vi "Init DaqEngine local AI SM.vi"(7 "AI TaskName":string, 8 "error in (no error)":errorcluster, 11 "DAQ Process AppData":T1) -> (0 "error out":errorcluster, 1 "local LoopCmdQ":refnum<queue>, 3 "DaqProces AI AppData+":T12)   [LabVIEW 2017, in "DAQ.lvclass"]
doc: "Developed by Kevin Thompson\nkevin@thompsonengineering.net\n\nCopyright 2018-2020\nThompson Engineering, LLC"
uses:
  DAQ.lvclass
  Process_DAQ SM AppData--cluster.ctl
  DataTypes/TD DAQ Settings--cluster.ctl
  DataTypes/TD DI Instrument Settings--cluster.ctl
  DataTypes/TD AI Instrument Settings--cluster.ctl
  DataTypes/TD AI InstSettings--cluster.ctl
  TD SimAI Ranges--cluster.ctl
  <vilib>/TELLC/Dynamic CVT API/TD Dynamic CVT DVR--ref.ctl
  DataTypes/TD AI local thread params--clustser.ctl
  Support/DataQueues/DataTypes/Analog DataSet MultiRow--QRef.ctl
  Support/DataQueues/DataTypes/Analog DataSet MultiRow--cluster.ctl
  Support/DataQueues/DataTypes/Analog DataSet MultiRow & ChanNames--QRef.ctl
  Support/DataQueues/DataTypes/Analog DataSet MultiRow & ChanNames--cluster.ctl
  DataTypes/TD AI TaskIO.ctl
  Support/DataQueues/DataTypes/DataQ SelectType--enum.ctl
  DAQ.lvclass/DAQ.ctl
  Accessors/Get DAQNodes Dict.vi
  Accessors/Get DAQ Settings.vi
  Accessors/Get Dependency.vi
  Get AI DAQ SMQ - single.vi
  Config/Config.lvclass
  Support/DataQueues/DataQueues.lvclass
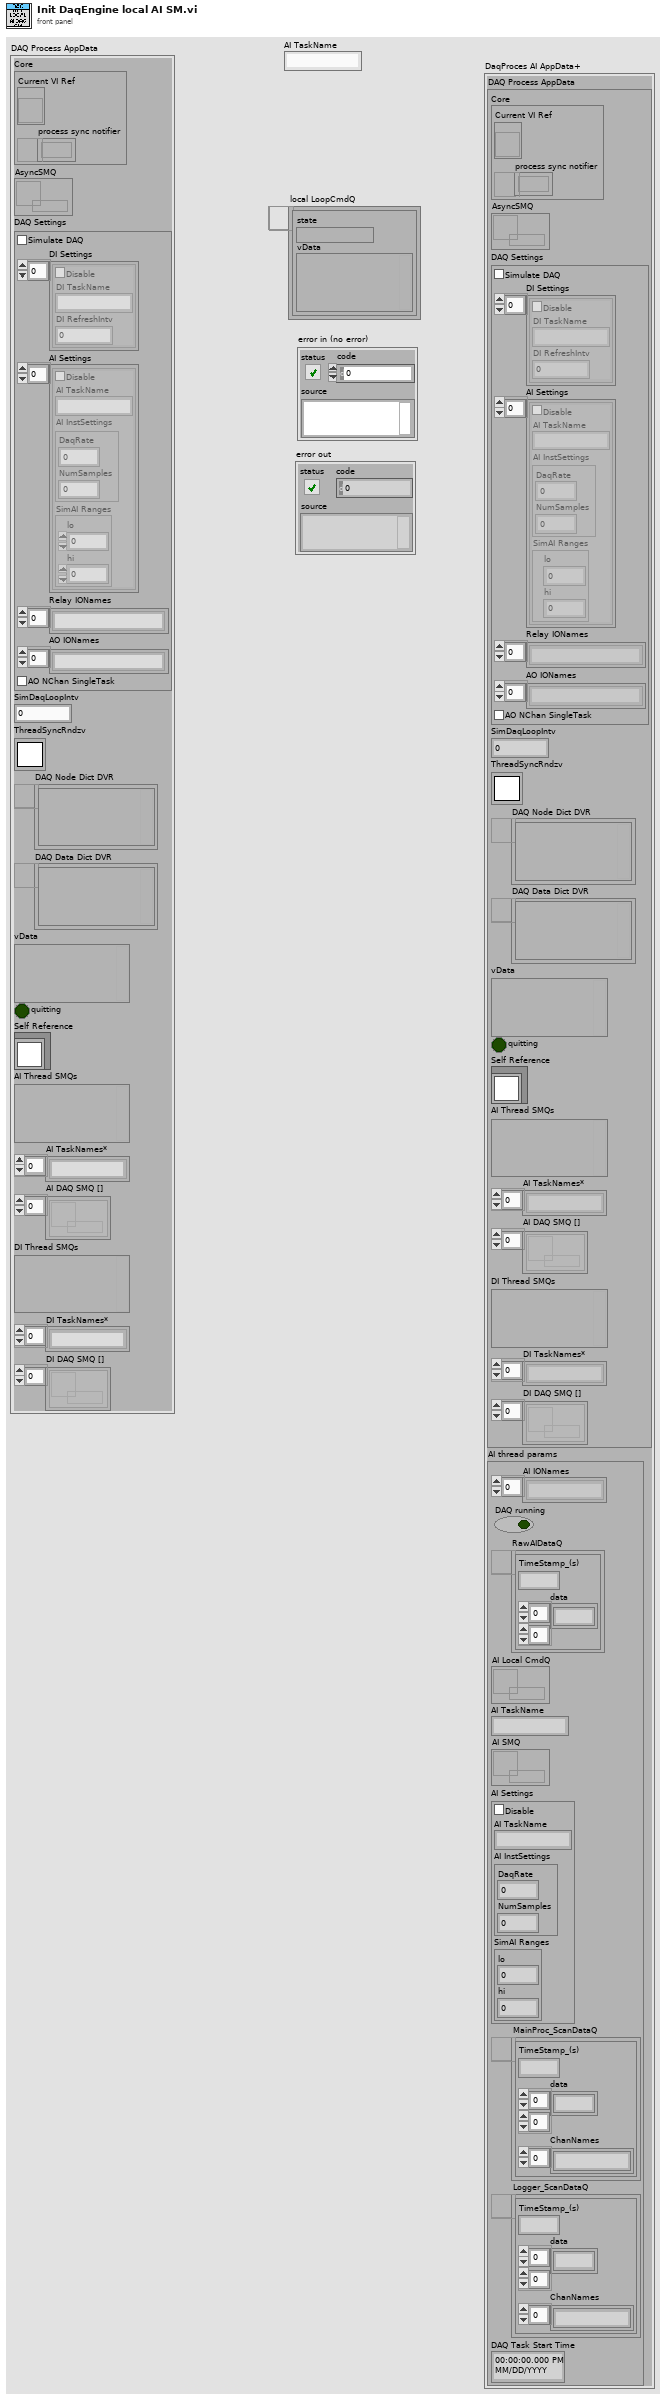
[diagram p1: front panel]
types:
  T1 = typedef "DAQ.lvclass/Process_DAQ SM AppData--cluster.ctl" = cluster{"Core":cluster{"Current VI Ref":refnum<vi>, "process sync notifier":refnum<notifier>}, "AsyncSMQ":refnum<queue>, "DAQ Settings":T2, "SimDaqLoopIntv":i32, "ThreadSyncRndzv":T7, "DAQ Node Dict DVR":T8, "DAQ Data Dict DVR":T8, "vData":variant, "quitting":bool, "Self Reference":refnum<class "DAQ.lvclass">, "AI Thread SMQs":variant, "AI TaskNames*":string[], "AI DAQ SMQ []":refnum<queue>[], "DI Thread SMQs":variant, "DI TaskNames*":string[], "DI DAQ SMQ []":refnum<queue>[]}
  T2 = typedef "DAQ.lvclass/TD DAQ Settings--cluster.ctl" = cluster{"Simulate DAQ":bool, "DI Settings":T3[], "AI Settings":T4[], "Relay IONames":string[], "AO IONames":string[], "AO NChan SingleTask":bool}
  T3 = typedef "DAQ.lvclass/TD DI Instrument Settings--cluster.ctl" = cluster{"Disable":bool, "DI TaskName":string, "DI RefreshIntv":i32}
  T4 = typedef "DAQ.lvclass/TD AI Instrument Settings--cluster.ctl" = cluster{"Disable":bool, "AI TaskName":string, "AI InstSettings":T5, "SimAI Ranges":T6}
  T5 = typedef "DAQ.lvclass/TD AI InstSettings--cluster.ctl" = cluster{"DaqRate":dbl, "NumSamples":i32}
  T6 = typedef "DAQ.lvclass/TD SimAI Ranges--cluster.ctl" = cluster{"lo":dbl, "hi":dbl}
  T7 = typedef "Rendezvous RefNum" = refnum<k1>
  T8 = typedef "TD Dynamic CVT DVR--ref.ctl" = refnum<data-value>
  T9 = typedef "DAQ.lvclass/TD AI local thread params--clustser.ctl" = cluster{"AI IONames":string[], "DAQ running":bool, "RawAIDataQ":T10, "AI Local CmdQ":refnum<queue>, "AI TaskName":string, "AI SMQ":refnum<queue>, "AI Settings":T4, "MainProc_ScanDataQ":T11, "Logger_ScanDataQ":T11, "DAQ Task Start Time":timestamp}
  T10 = typedef "DataQueues.lvclass/Analog DataSet MultiRow--QRef.ctl" = refnum<queue>
  T11 = typedef "DataQueues.lvclass/Analog DataSet MultiRow & ChanNames--QRef.ctl" = refnum<queue>
  T12 = cluster{"DAQ Process AppData":T1, "AI thread params":T9}
  T13 = typedef "DataQueues.lvclass/DataQ SelectType--enum.ctl" = enum16{"MainProcess", "LogEngine", "LocalDAQThread"}
  T14 = typedef "DAQ.lvclass/TD AI TaskIO.ctl" = cluster{"AI TaskName":string, "IONames":string[], "DAQmx AI TaskRef":refnum<k21>}
  T15 = typedef "DAQ.lvclass/Dependency--cluster.ctl" = cluster{"Config":refnum<class "Config.lvclass">, "DataQueues":refnum<class "DataQueues.lvclass">}
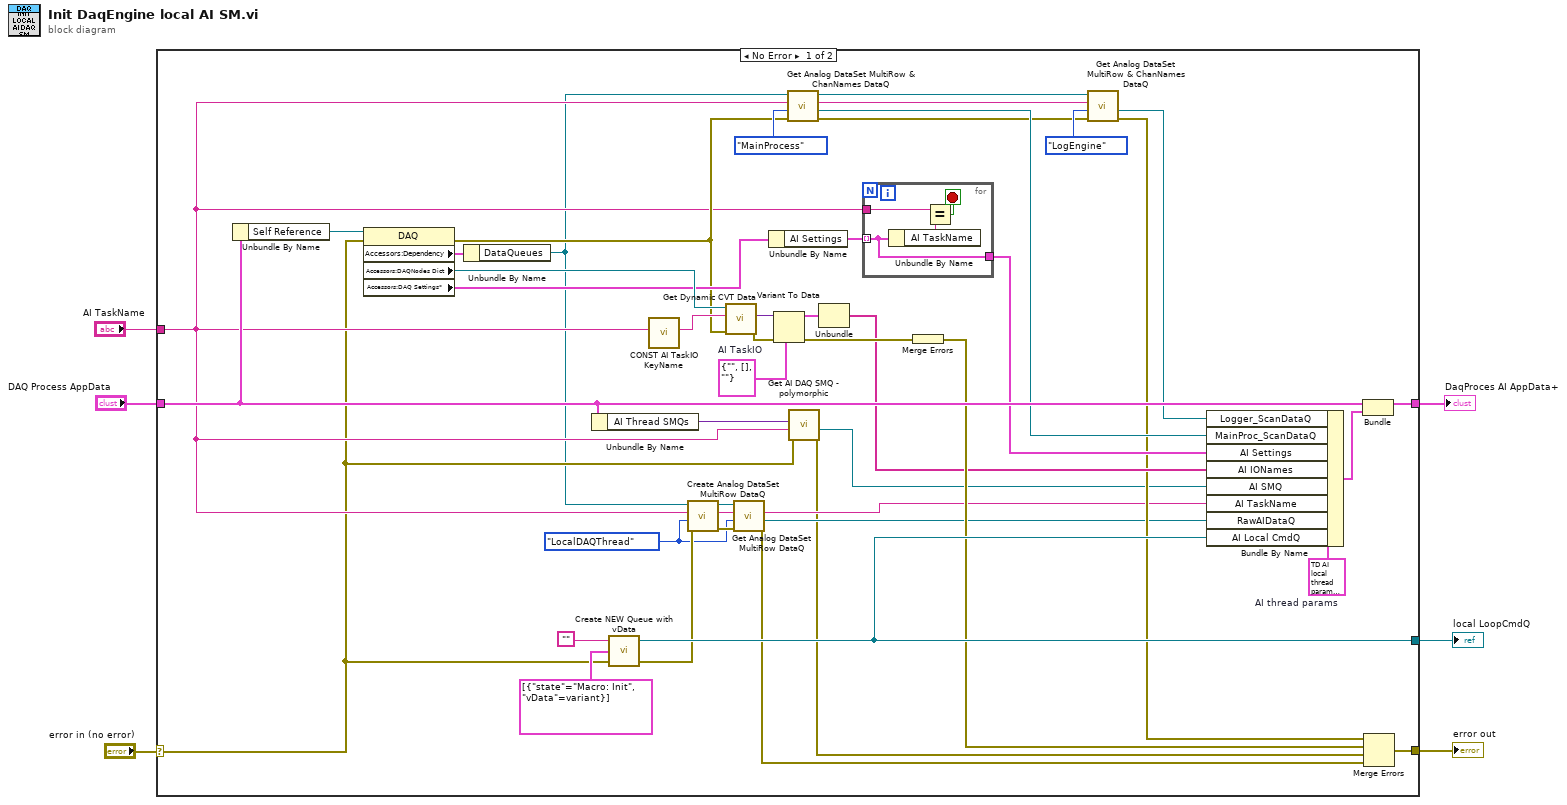
[diagram p0: block diagram]
diagram:
  n1 = case shown="No Error" "error in (no error)" {
    selector: "error in (no error)" -> [w11 w56]
    tunnel: "DAQ Process AppData" -> [w40 _]
    tunnel: [w47 _] -> w6
    tunnel: [w49 _] -> w3
    tunnel: [w50 w56] -> w5
    tunnel: "AI TaskName" -> [w13 _]
    frame No Error {
      w9 = DataQ_SelectType--enum."LocalDAQThread" ("Select")
      w32 = T14 {"AI TaskName"="", "IONames"=[], "DAQmx AI TaskRef"=""}  # AI TaskIO
      w48 = T9 {"AI IONames"=[], "DAQ running"=FALSE, "RawAIDataQ"=refnum, "AI Local CmdQ"=refnum, "AI TaskName"="", "AI SMQ"=refnum, "AI Settings"={"Disable"=FALSE, "AI TaskName"="", "AI InstSettings"={"DaqRate"=0.0, "NumSamples"=0}, "SimAI Ranges"={"lo"=0.0, "hi"=0.0}}, "MainProc_ScanDataQ"=refnum, "Logger_ScanDataQ"=refnum, "DAQ Task Start Time"=timestamp(0 s since 1904-01-01)}  # AI thread params
      n2 = Unbundle By Name(w40) -> ("Self Reference"=w46:refnum<class "DAQ.lvclass">)
      n3 = property class="DAQ"(reference=w46, error in=w11) -> (error out=w30:errorcluster, "Accessors:Dependency"=w8:T15, "Accessors:DAQNodes Dict"=w36:T8, "Accessors:DAQ Settings*"=w33:T2)  [unwired: 1 out]
      n4 = Unbundle By Name(w8) -> ("DataQueues"=w7:refnum<class "DataQueues.lvclass">)
      n5 = Unbundle By Name(w40) -> ("AI Thread SMQs"=w14:variant)
      n6 = call <vilib>:"Create NEW Queue with vData.vi"("error in (no error)"=w11, "Initial States"=cluster{"state":string, "vData":variant}[] [{"state"="Macro: Init", "vData"=variant}], "Name (SMQ)"="") -> ("error out"=w15:errorcluster, "queue out"=w47:refnum<queue>)  [unwired: 1 in]
      n7 = call "CONST AI TaskIO KeyName.vi"("AI TaskName"=w13) -> ("AI TaskIO (KeyName)"=w45:string)  [unwired: 10 in]
      n8 = call "Create Analog DataSet MultiRow DataQ.vi"("error in (no error)"=w15, "Select"=w9, "TaskName"=w13, "DataQueues in"=w7) -> ("error out"=w17:errorcluster, "TaskName out"=w18:string, "DataQueues out"=w16:refnum<class "DataQueues.lvclass">)  [unwired: 5 in]
      n9 = call <vilib>:"Get Dynamic CVT Data.vi"("error in (no error)"=w30, "DataName"=w45, "dCVT DVR"=w36) -> ("error out"=w43:errorcluster, "value"=w44:variant)  [unwired: 5 in, 2 out]
      n10 = call "Get Analog DataSet MultiRow DataQ.vi"("error in (no error)"=w17, "Select"=w9, "TaskName"=w18, "DataQueues in"=w16) -> ("error out"=w20:errorcluster, "Analog DataSet MultiRow QRef"=w21:T10, "TaskName out"=w19:string)  [unwired: 3 in, 2 out]
      n11 = Unbundle By Name(w33) -> ("AI Settings"=w39:T4[])
      n12 = Variant To Data(error in=w43, type=w32, Variant=w44) -> (data=w35:T14, error out=w42:errorcluster)
      n13 = call "Get Analog DataSet MultiRow & ChanNames DataQ.vi"("error in (no error)"=w30, "Select"=DataQ_SelectType--enum."MainProcess", "TaskName"=w13, "DataQueues in"=w7) -> ("error out"=w23:errorcluster, "Analog DataSet MultiRow & ChanNames QRef"=w29:T11, "TaskName out"=w26:string, "DataQueues out"=w27:refnum<class "DataQueues.lvclass">)  [unwired: 3 in, 1 out]
      n14 = call-poly "Get AI DAQ SMQ - polymorphic.vi"("error in (no error)"=w11, "AI TaskName"=w13, "AI Thread SMQs"=w14) -> ("error out"=w10:errorcluster, "AI DAQ SMQ"=w12:refnum<queue>)  [unwired: 6 in, 1 out]
      n15 = Unbundle(w35) -> ("IONames"=w34:string[])  [unwired: 2 out]
      n16 = for {
        tunnel: w39 -> [w52] mode=indexing
        tunnel: w13 -> [w55]
        tunnel: [w52] -> w38
        stop <- w53 stop-if-true
        n17 = Unbundle By Name(w52) -> ("AI TaskName"=w54:string)
        n18 = Equal?(x=w55, y=w54) -> (x = y?=w53:bool)
      }
      n19 = Merge Errors(w42) -> (w37:errorcluster)
      n20 = call "Get Analog DataSet MultiRow & ChanNames DataQ.vi"("error in (no error)"=w23, "Select"=DataQ_SelectType--enum."LogEngine", "TaskName"=w26, "DataQueues in"=w27) -> ("error out"=w22:errorcluster, "Analog DataSet MultiRow & ChanNames QRef"=w24:T11)  [unwired: 3 in, 3 out]
      n21 = Bundle By Name(cluster=w48, "Logger_ScanDataQ"=w24, "MainProc_ScanDataQ"=w29, "AI Settings"=w38, "AI IONames"=w34, "AI SMQ"=w12, "AI TaskName"=w19, "RawAIDataQ"=w21, "AI Local CmdQ"=w47) -> (w25:T9)
      n22 = Bundle("DAQ Process AppData"=w40, "AI thread params"=w25) -> (w49:T12)  [unwired: 1 in]
      n23 = Merge Errors(w22, w37, w10, w20) -> (w50:errorcluster)
    }
    frame Error {
    }
  }
  "error out" <- w5
  "local LoopCmdQ" <- w6
  "DaqProces AI AppData+" <- w3
